vi "_CSMObj-Obtain CSMObj.vi"(7 "Allowed Messages(Empty for all)":string[](array[string]), 8 "error in (no error)":errorcluster, 11 "Requested Name":string) -> (0 "error out":errorcluster, 3 "CSMQ out":T1)   [LabVIEW 2017, in "Communicable State Machine.lvlib"]
uses:
  Communicable State Machine.lvlib
  _CSMObj.ctl
  Priority Queue/Priority Queue.lvclass
  Typedef/_CSM_MODE.ctl
  _CSMObj-Data.ctl
  Typedef/_CSM Status Change Event Data.ctl
  _CSMObj-ModeData.ctl
  Priority Queue/Priority Queue.lvclass/Priority Queue.ctl
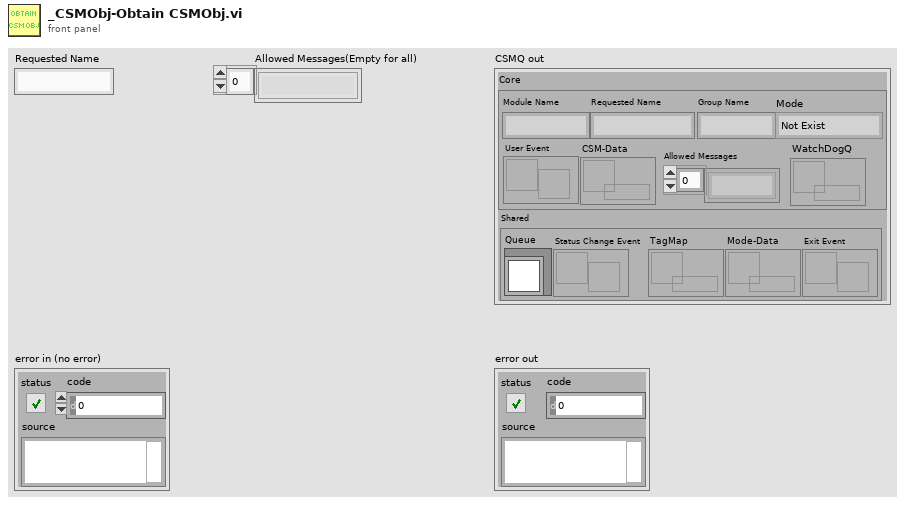
[diagram p1: front panel]
types:
  T1 = typedef "Communicable State Machine.lvlib/_CSMObj.ctl" = cluster{"Core":cluster{"Module Name":string, "Requested Name":string, "Group Name":string, "Mode":T2, "User Event":refnum<user-event>, "CSM-Data":refnum<data-value>, "Allowed Messages":string[], "WatchDogQ":refnum<queue>}, "Shared":cluster{"Queue":refnum<class "Priority Queue.lvclass">, "Status Change Event":refnum<user-event>, "TagMap":refnum<data-value>, "Mode-Data":refnum<data-value>, "Exit Event":refnum<user-event>}}
  T2 = typedef "Communicable State Machine.lvlib/_CSM_MODE.ctl" = enum16{"Not Exist", "Stand Alone", "CSM", "Worker", "Worker Agent", "Chain Node", "Chain"}
  T3 = typedef "Communicable State Machine.lvlib/_CSMObj-ModeData.ctl" = cluster{"CSMDataDVR":refnum<data-value>[], "Messages of Chain Nodes":cluster{"Module Name":string, "Allowed Messages":string[]}[], "Chain Message Mapping Map":variant}
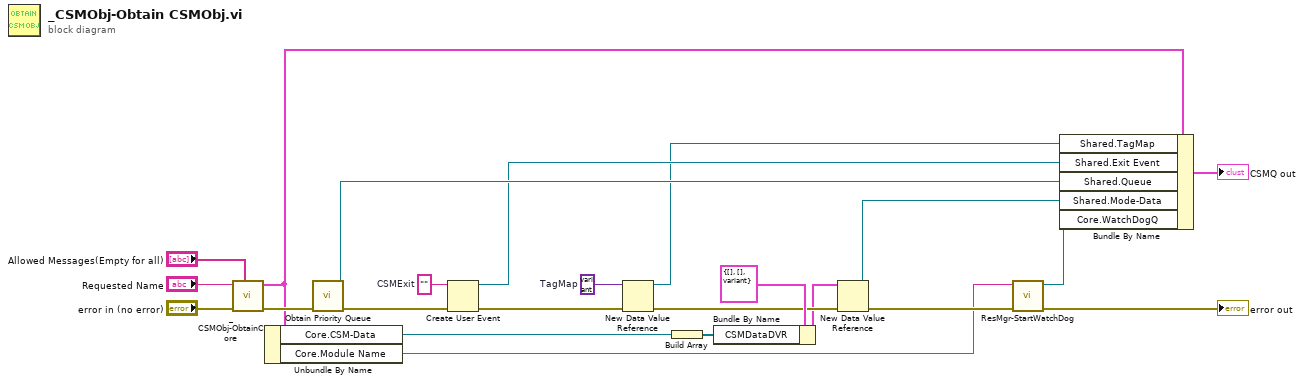
[diagram p0: block diagram]
diagram:
  w15 = variant  # TagMap
  w16 = ""  # CSMExit
  n1 = call "_CSMObj-ObtainCore.vi"("Allowed Messages(Empty for all)"="Allowed Messages(Empty for all)", "Error in"="error in (no error)", "Requested Name"="Requested Name") -> ("Error out"=w23:errorcluster, "CSMQ out"=w7:T1)  [unwired: 7 in]
  n2 = Unbundle By Name(w7) -> ("Core.CSM-Data"=w6:refnum<data-value>, "Core.Module Name"=w1:string)
  n3 = call "Obtain Priority Queue.vi"("error in (no error)"=w23) -> ("error out"=w18:errorcluster, "Priority Queue"=w14:refnum<class "Priority Queue.lvclass">)  [unwired: 8 in, 1 out]
  n4 = Create User Event(user event datatype=w16, error in=w18) -> (user event=w13:refnum<user-event>, error out=w17:errorcluster)
  n5 = New Data Value Reference(data value=w15, error in=w17) -> (data value reference=w12:refnum<data-value>, error out=w10:errorcluster)
  n6 = Build Array(w6) -> (w5:refnum<data-value>[])
  n7 = Bundle By Name(cluster=T3 {"CSMDataDVR"=[], "Messages of Chain Nodes"=[], "Chain Message Mapping Map"=variant} ("CSMObj-Data"), "CSMDataDVR"=w5) -> (w8:T3)
  n8 = New Data Value Reference(data value=w8, error in=w10) -> (data value reference=w9:refnum<data-value>, error out=w4:errorcluster)
  n9 = call "ResMgr-StartWatchDog.vi"("error in (no error)"=w4, "ModuleName"=w1) -> ("error out"=→"error out":errorcluster, "WatchDogQ"=w2:refnum<queue>)  [unwired: 8 in]
  n10 = Bundle By Name(cluster=w7, "Shared.TagMap"=w12, "Shared.Exit Event"=w13, "Shared.Queue"=w14, "Shared.Mode-Data"=w9, "Core.WatchDogQ"=w2) -> (→"CSMQ out":T1)
